vi "writeNewQBdata.vi"(8 "error in (no error)":errorcluster, 9 "newQBdata":string[][](array[string]), 10 "path":path) -> (0 "error out":errorcluster, 2 "Refnum Cluster Out":T1)   [LabVIEW 2012]
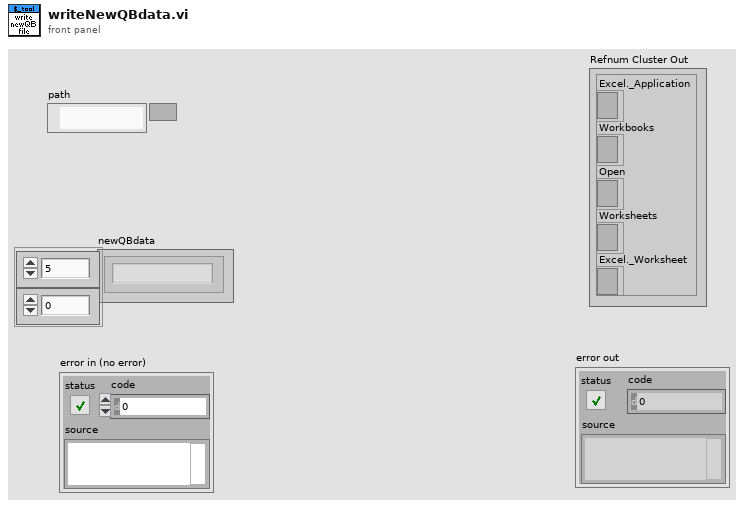
[diagram p1: front panel]
types:
  T1 = cluster{"Excel._Application":refnum<k7>, "Workbooks":refnum<k7>, "Open":refnum<k7>, "Worksheets":refnum<k7>, "Excel._Worksheet":refnum<k7>}
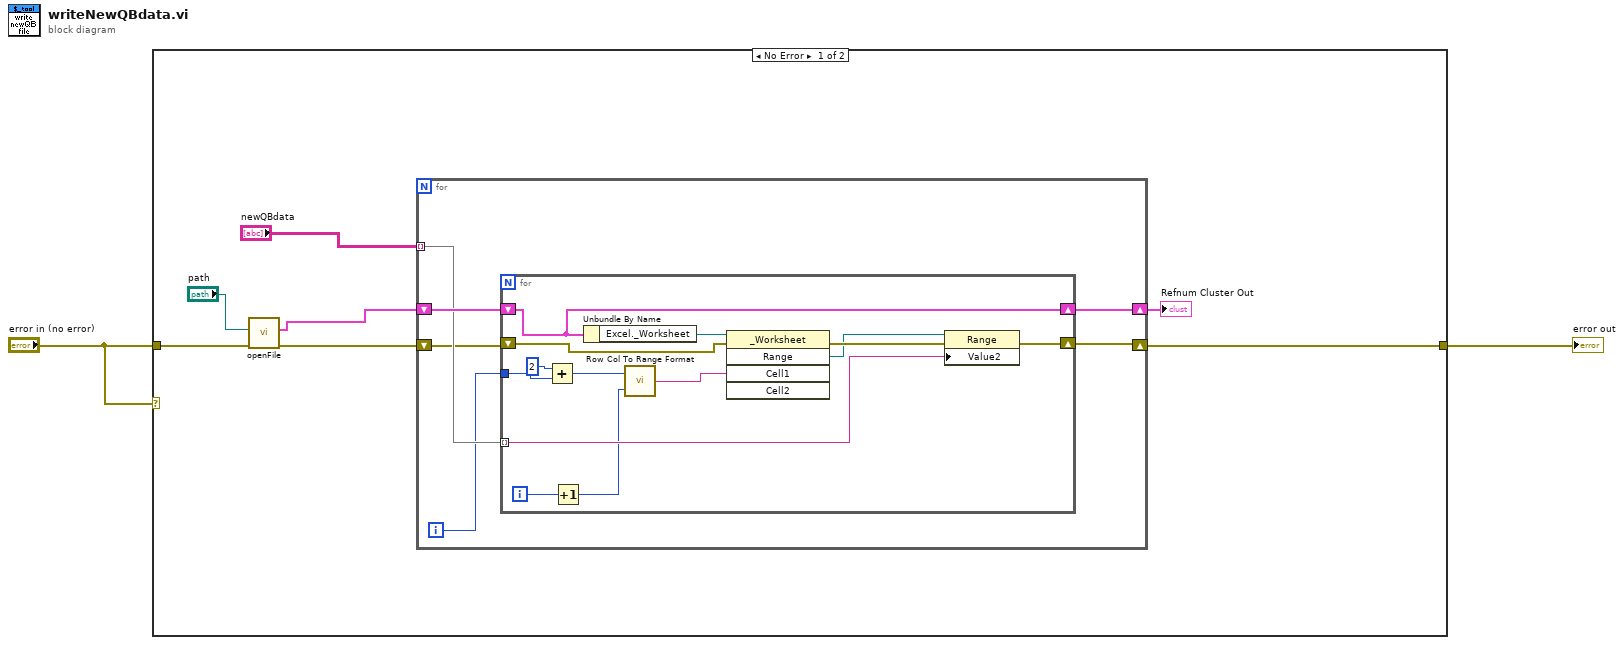
[diagram p0: block diagram]
diagram:
  n1 = case shown="No Error" "error in (no error)" {
    tunnel: "error in (no error)" -> [w8 w29]
    tunnel: [w4 w29] -> w2
    frame No Error {
      n2 = call "openFile.vi"("error in (no error)"=w8, "path"="path") -> ("error out"=w7:errorcluster, "Refnum Cluster Out"=w5:T1)  [unwired: 8 in]
      n3 = for {
        tunnel: "newQBdata" -> [w14] mode=indexing
        shift-right: [w12] -> w3
        shift-left: w5 -> [w15]
        shift-right: [w11] -> w4
        shift-left: w7 -> [w10]
        i -> [w13]
        n4 = for {
          tunnel: w14 -> [w25] mode=indexing
          tunnel: w13 -> [w23]
          shift-right: [w22] -> w12
          shift-left: w15 -> [w22]
          shift-right: [w21] -> w11
          shift-left: w10 -> [w20]
          i -> [w24]
          n5 = Add(x=2, y=w23) -> (x+y=w19:i32)
          n6 = Increment(x=w24) -> (x+1=w18:i32)
          n7 = Unbundle By Name(w22) -> ("Excel._Worksheet"=w16:refnum<k7>)
          n8 = call <userlib>:"Row Col To Range Format.vi"("Column"=w18, "Row"=w19) -> ("Output String"=w28:string)
          n9 = invoke class="_Worksheet" method="Range"(reference=w16, error in=w20, "Cell1"=w28) -> (error out=w27:errorcluster, "Range"=w26:refnum<k7>)  [unwired: 2 in, 3 out]
          n10 = property class="Range"(reference=w26, error in=w27, "Value2"=w25) -> (error out=w21:errorcluster)  [unwired: 1 out]
        }
      }
      "Refnum Cluster Out" <- w3
    }
    frame Error {
    }
  }
  "error out" <- w2
